vi "Easy Style Setup.vi"(4 "font style (regular)":T1(ring), 6 "font Size(9)":sgl=9.0, 8 "error in (no error)":errorcluster, 9 "Alignment":i32(ring)=1 items=["NotSet"=0, "TopLeft"=1, "TopCenter"=2, "TopRight"=4, "MiddleLeft"=16, "MiddleCenter"=32, "MiddleRight"=64, "BottomLeft"=256, "BottomCenter"=512, "BottomRight"=1024], 10 "Color BG":u32(colorbox)=14474460, 11 "Color FG":u32(colorbox)) -> (0 "error out":errorcluster, 2 "CellStyle out":refnum<class "CellStyle.lvclass">)   [LabVIEW 2014]
doc: "Quick access to easily setup a style, used to format a cell or specific cell type. Color is required, where others are optional settings. More detailed style, colors and fonts are available in the specific classes and the .net style properties themselves."
uses:
  CellStyle/CellStyle.lvclass
  CellStyle/CellStyleCluster.ctl
  Color/Color.lvclass
  Font/Font.lvclass
  Font/Font Cluster.ctl
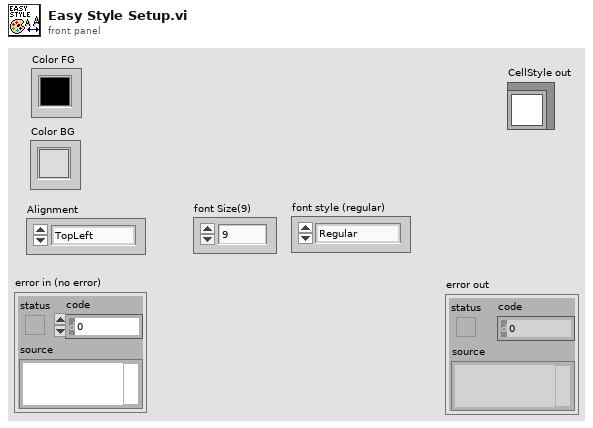
[diagram p1: front panel]
types:
  T1 = enum16{"Regular", "Bold", "Italic", "Underline", "Strikeout"}
  T2 = typedef "Font.lvclass/Font Cluster.ctl" = cluster{"familyName":string, "emSize":sgl, "style":enum16{"Regular", "Bold", "Italic", "Underline", "Strikeout"}}
  T3 = typedef "CellStyle.lvclass/CellStyleCluster.ctl" = cluster{"Alignment":i32, "WrapMode":i32, "ForeColor":refnum<class "Color.lvclass">, "SelectionForeColor":refnum<class "Color.lvclass">, "BackColor":refnum<class "Color.lvclass">, "SelectionBackColor":refnum<class "Color.lvclass">, "Font":refnum<class "Font.lvclass">}
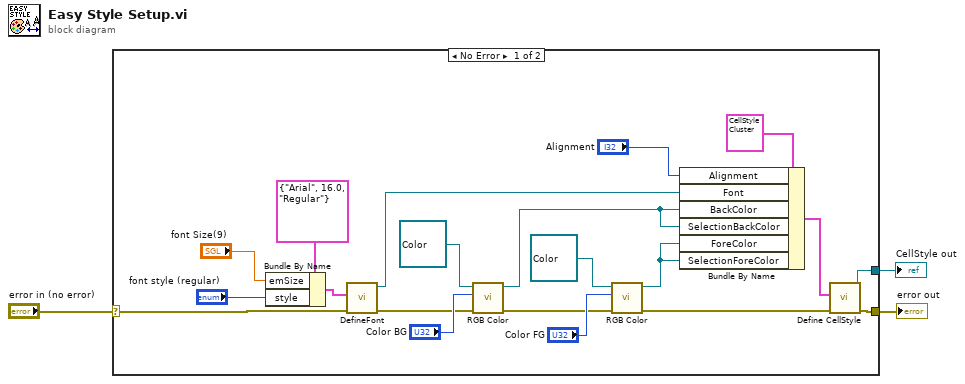
[diagram p0: block diagram]
diagram:
  n1 = case shown="No Error" "error in (no error)" {
    selector: "error in (no error)" -> [w8 w24]
    tunnel: [w9 w24] -> w3
    tunnel: [w4 _] -> w1
    frame No Error {
      n2 = Bundle By Name(cluster=T2 {"familyName"="Arial", "emSize"=16.0, "style"=enum."Regular"} ("Font Cluster"), "emSize"="font Size(9)", "style"="font style (regular)") -> (w15:T2)
      n3 = call "DefineFont.vi"("error in (no error)"=w8, "Font Cluster"=w15) -> ("error out"=w12:errorcluster, "Font out"=w5:refnum<class "Font.lvclass">)  [unwired: 8 in]
      n4 = call-dynamic "RGB Color.vi"("error in (no error)"=w12, "Color"="Color BG", "Color in"=refnum<class "Color.lvclass"> refnum ("Color.lvclass")) -> ("error out"=w11:errorcluster, "Color out"=w6:refnum<class "Color.lvclass">)  [unwired: 7 in]
      n5 = call-dynamic "RGB Color.vi"("error in (no error)"=w11, "Color"="Color FG", "Color in"=refnum<class "Color.lvclass"> refnum ("Color.lvclass")) -> ("error out"=w10:errorcluster, "Color out"=w19:refnum<class "Color.lvclass">)  [unwired: 7 in]
      n6 = Bundle By Name(cluster=T3 {"Alignment"=2, "WrapMode"=1, "ForeColor"=refnum, "SelectionForeColor"=refnum, "BackColor"=refnum, "SelectionBackColor"=refnum, "Font"=refnum} ("CellStyle"), "Alignment"="Alignment", "Font"=w5, "BackColor"=w6, "SelectionBackColor"=w6, "ForeColor"=w19, "SelectionForeColor"=w19) -> (w22:T3)
      n7 = call "Define CellStyle.vi"("error in (no error)"=w10, "CellStyle"=w22) -> ("error out"=w9:errorcluster, "CellStyle out"=w4:refnum<class "CellStyle.lvclass">)  [unwired: 8 in]
    }
    frame Error {
    }
  }
  "error out" <- w3
  "CellStyle out" <- w1
